vi "TestStand_Control ( Configure_Application_Manager ).vi"(8 "error IO":errorcluster, 11 "TestStand UI Data":T1) -> (0 "error IO 2":errorcluster, 3 "TestStand UI Data 2":T1)   [LabVIEW 2018, in "TestStand_Control.lvlib"]
uses:
  TestStand_Control.lvlib
  Module_Controls/TestStand UI Data.ctl
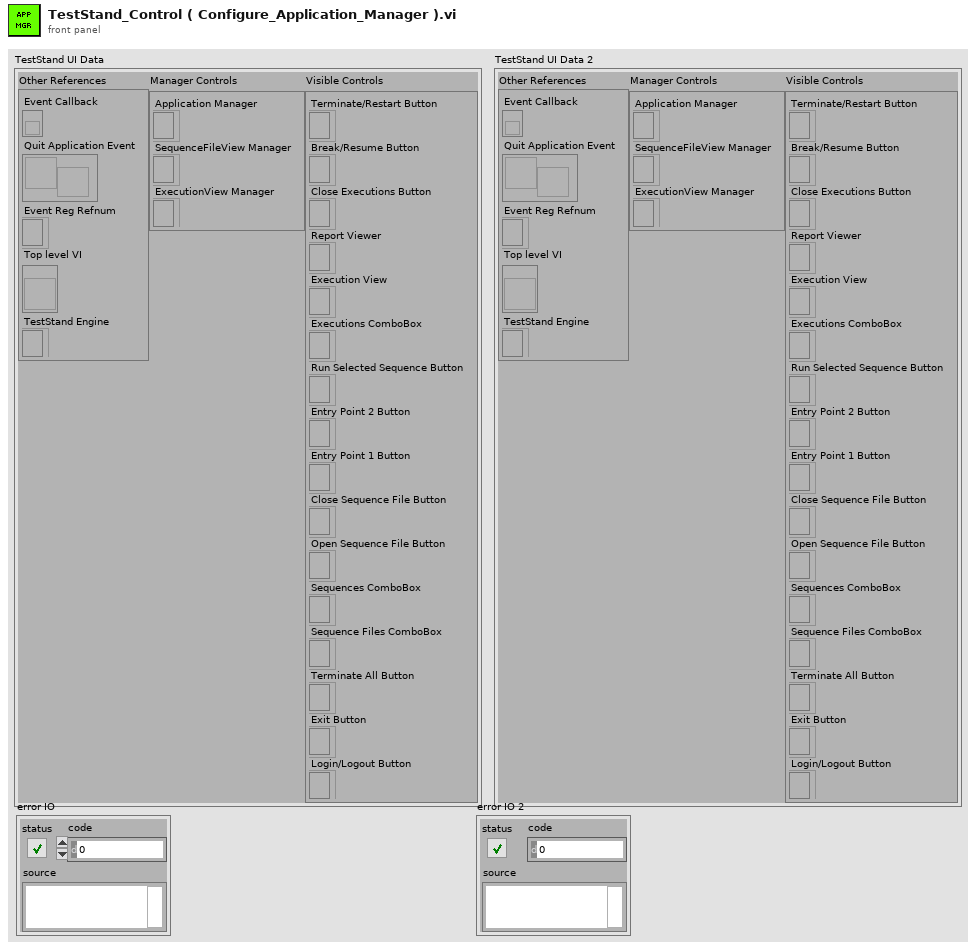
[diagram p1: front panel]
types:
  T1 = typedef "TestStand_Control.lvlib/TestStand UI Data.ctl" = cluster{"Other References":cluster{"Event Callback":refnum<k27>, "Quit Application Event":refnum<user-event>, "Event Reg Refnum":refnum<event-registration>, "Top level VI":refnum<vi>, "TestStand Engine":refnum<k7>}, "Manager Controls":cluster{"Application Manager":refnum<k7>, "SequenceFileView Manager":refnum<k7>, "ExecutionView Manager":refnum<k7>}, "Visible Controls":cluster{"Terminate/Restart Button":refnum<k7>, "Break/Resume Button":refnum<k7>, "Close Executions Button":refnum<k7>, "Report Viewer":refnum<k7>, "Execution View":refnum<k7>, "Executions ComboBox":refnum<k7>, "Run Selected Sequence Button":refnum<k7>, "Entry Point 2 Button":refnum<k7>, "Entry Point 1 Button":refnum<k7>, "Close Sequence File Button":refnum<k7>, "Open Sequence File Button":refnum<k7>, "Sequences ComboBox":refnum<k7>, "Sequence Files ComboBox":refnum<k7>, "Terminate All Button":refnum<k7>, "Exit Button":refnum<k7>, "Login/Logout Button":refnum<k7>}}
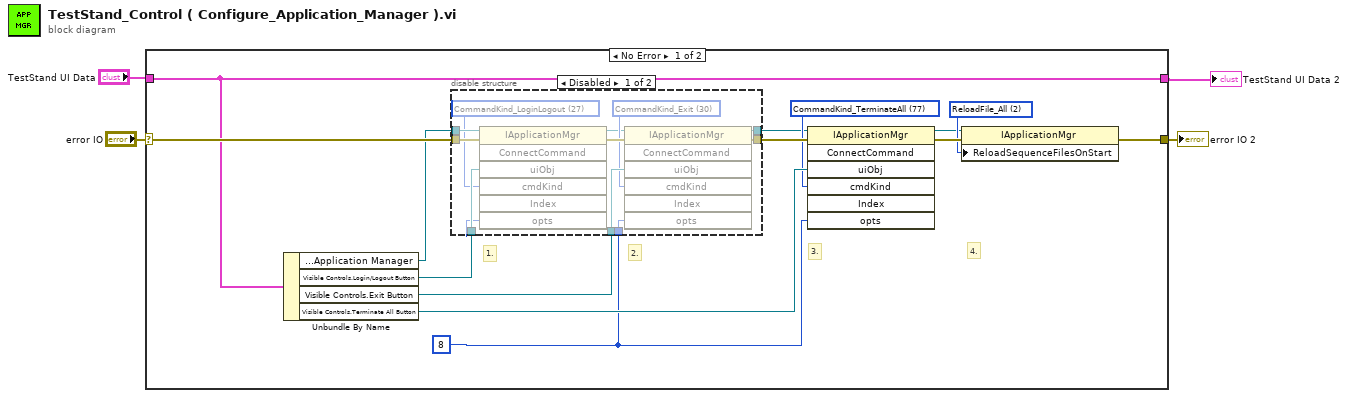
[diagram p0: block diagram]
diagram:
  n1 = case shown="No Error" "error IO" {
    selector: "error IO" -> [w18 w33]
    tunnel: [w12 w33] -> w1
    tunnel: "TestStand UI Data" -> [w9 w32]
    tunnel: [w9 w32] -> w3
    frame No Error {
      w6 = 77 items=["CommandKind_NotACommand"=0, "CommandKind_Container"=1, "CommandKind_Separator"=2, "CommandKind_Custom"=3, "CommandKind_OpenSequenceFile"=20, "CommandKind_Close"=21, "CommandKind_CloseAll"=22, "CommandKind_CloseCompletedExecutions"=23, "CommandKind_OpenWorkspaceBrowser"=24, "CommandKind_Login"=25, "CommandKind_Logout"=26, "CommandKind_LoginLogout"=27, "CommandKind_UnloadAllModules"=28, "CommandKind_MRUFile"=29, "CommandKind_Exit"=30, "CommandKind_Restart"=40, "CommandKind_RunEntryPoint"=41, "CommandKind_RunEntryPointOnSelectedSteps"=42, "CommandKind_LoopEntryPointOnSelectedSteps"=43, "CommandKind_RunCurrentSequence"=44, "CommandKind_RunSpecificSequence"=45, "CommandKind_RunSelectedSteps"=46, "CommandKind_RunSelectedStepsUsingEntryPointsSubmenu"=47, "CommandKind_LoopOnSelectedSteps"=48, "CommandKind_LoopOnSelectedStepsUsingEntryPointsSubmenu"=49, "CommandKind_BreakOnFirstStep"=50, "CommandKind_BreakOnStepFailure"=51, "CommandKind_BreakOnSequenceFailure"=52, "CommandKind_TracingEnabled"=53, "CommandKind_ToggleBreakpoint"=60, "CommandKind_SetRunModeSubmenu"=61, "CommandKind_RunModeForcePass"=62, "CommandKind_RunModeForceFail"=63, "CommandKind_RunModeSkip"=64, "CommandKind_RunModeNormal"=65, "CommandKind_Resume"=66, "CommandKind_StepInto"=67, "CommandKind_StepOver"=68, "CommandKind_StepOut"=69, "CommandKind_SetNextStep"=70, "CommandKind_Break"=71, "CommandKind_BreakResume"=72, "CommandKind_Terminate"=73, "CommandKind_TerminateRestart"=74, "CommandKind_Abort"=75, "CommandKind_BreakAll"=76, "CommandKind_TerminateAll"=77, "CommandKind_AbortAll"=78, "CommandKind_ResumeAll"=79, "CommandKind_DisplayBreakpointsAndWatchExpressions"=80, "CommandKind_DisplayBreakpointSettings"=81, "CommandKind_BreakpointSubmenu"=85, "CommandKind_ConfigureAdapters"=90, "CommandKind_ConfigureStationOptions"=91, "CommandKind_ConfigureSearchDirectories"=92, "CommandKind_ConfigureExternalViewers"=93, "CommandKind_ToolItem"=100, "CommandKind_CustomizeTools"=101, "CommandKind_ExecutionEntryPointInsertionMarker"=110, "CommandKind_ExecutionEntryPointDefaultMenuInsertionMarker"=111, "CommandKind_ConfigurationEntryPointInsertionMarker"=112, "CommandKind_ConfigurationEntryPointDefaultMenuInsertionMarker"=113, "CommandKind_DefaultFileMenu_Set"=120, "CommandKind_DefaultExecuteMenu_Set"=121, "CommandKind_DefaultDebugMenu_Set"=123, "CommandKind_DefaultConfigureMenu_Set"=124, "CommandKind_DefaultToolsMenu_Set"=125, "CommandKind_DefaultSequenceViewContextMenu_Set"=126, "CommandKind_DefaultListBarContextMenu_Set"=127, "CommandKind_MRUFiles_Set"=140, "CommandKind_ExecutionEntryPoints_Set"=141, "CommandKind_RunSequences_Set"=142, "CommandKind_RunSelectedStepsUsingEntryPoints_Set"=143, "CommandKind_LoopOnSelectedStepsUsingEntryPoints_Set"=144, "CommandKind_ConfigurationEntryPoints_Set"=145, "CommandKind_Tools_Set"=146] ("cmdKind")
      w8 = 8 ("opts")
      w13 = 2 items=["ReloadFile_None", "ReloadFile_Selected", "ReloadFile_All"] ("ReloadSequenceFilesOnStart")
      # "4."
      # "3."
      # "2."
      # "1."
      n2 = Unbundle By Name(w9) -> ("Manager Controls.Application Manager"=w11:refnum<k7>, "Visible Controls.Login/Logout Button"=w17:refnum<k7>, "Visible Controls.Exit Button"=w16:refnum<k7>, "Visible Controls.Terminate All Button"=w15:refnum<k7>)
      n3 = disable-structure shown="Disabled" {
        disable-tunnel: w18 -> [w29 w30]
        disable-tunnel: w17 -> [w28 _]
        disable-tunnel: w16 -> [w27 _]
        disable-tunnel: w11 -> [w26 w31]
        disable-tunnel: w8 -> [w25 _]
        disable-tunnel: [w23 w30] -> w7
        disable-tunnel: [w20 w31] -> w5
        frame Disabled {
          w21 = 30 items=["CommandKind_NotACommand"=0, "CommandKind_Container"=1, "CommandKind_Separator"=2, "CommandKind_Custom"=3, "CommandKind_OpenSequenceFile"=20, "CommandKind_Close"=21, "CommandKind_CloseAll"=22, "CommandKind_CloseCompletedExecutions"=23, "CommandKind_OpenWorkspaceBrowser"=24, "CommandKind_Login"=25, "CommandKind_Logout"=26, "CommandKind_LoginLogout"=27, "CommandKind_UnloadAllModules"=28, "CommandKind_MRUFile"=29, "CommandKind_Exit"=30, "CommandKind_Restart"=40, "CommandKind_RunEntryPoint"=41, "CommandKind_RunEntryPointOnSelectedSteps"=42, "CommandKind_LoopEntryPointOnSelectedSteps"=43, "CommandKind_RunCurrentSequence"=44, "CommandKind_RunSpecificSequence"=45, "CommandKind_RunSelectedSteps"=46, "CommandKind_RunSelectedStepsUsingEntryPointsSubmenu"=47, "CommandKind_LoopOnSelectedSteps"=48, "CommandKind_LoopOnSelectedStepsUsingEntryPointsSubmenu"=49, "CommandKind_BreakOnFirstStep"=50, "CommandKind_BreakOnStepFailure"=51, "CommandKind_BreakOnSequenceFailure"=52, "CommandKind_TracingEnabled"=53, "CommandKind_ToggleBreakpoint"=60, "CommandKind_SetRunModeSubmenu"=61, "CommandKind_RunModeForcePass"=62, "CommandKind_RunModeForceFail"=63, "CommandKind_RunModeSkip"=64, "CommandKind_RunModeNormal"=65, "CommandKind_Resume"=66, "CommandKind_StepInto"=67, "CommandKind_StepOver"=68, "CommandKind_StepOut"=69, "CommandKind_SetNextStep"=70, "CommandKind_Break"=71, "CommandKind_BreakResume"=72, "CommandKind_Terminate"=73, "CommandKind_TerminateRestart"=74, "CommandKind_Abort"=75, "CommandKind_BreakAll"=76, "CommandKind_TerminateAll"=77, "CommandKind_AbortAll"=78, "CommandKind_ResumeAll"=79, "CommandKind_DisplayBreakpointsAndWatchExpressions"=80, "CommandKind_DisplayBreakpointSettings"=81, "CommandKind_BreakpointSubmenu"=85, "CommandKind_ConfigureAdapters"=90, "CommandKind_ConfigureStationOptions"=91, "CommandKind_ConfigureSearchDirectories"=92, "CommandKind_ConfigureExternalViewers"=93, "CommandKind_ToolItem"=100, "CommandKind_CustomizeTools"=101, "CommandKind_ExecutionEntryPointInsertionMarker"=110, "CommandKind_ExecutionEntryPointDefaultMenuInsertionMarker"=111, "CommandKind_ConfigurationEntryPointInsertionMarker"=112, "CommandKind_ConfigurationEntryPointDefaultMenuInsertionMarker"=113, "CommandKind_DefaultFileMenu_Set"=120, "CommandKind_DefaultExecuteMenu_Set"=121, "CommandKind_DefaultDebugMenu_Set"=123, "CommandKind_DefaultConfigureMenu_Set"=124, "CommandKind_DefaultToolsMenu_Set"=125, "CommandKind_DefaultSequenceViewContextMenu_Set"=126, "CommandKind_DefaultListBarContextMenu_Set"=127, "CommandKind_MRUFiles_Set"=140, "CommandKind_ExecutionEntryPoints_Set"=141, "CommandKind_RunSequences_Set"=142, "CommandKind_RunSelectedStepsUsingEntryPoints_Set"=143, "CommandKind_LoopOnSelectedStepsUsingEntryPoints_Set"=144, "CommandKind_ConfigurationEntryPoints_Set"=145, "CommandKind_Tools_Set"=146] ("cmdKind")
          w22 = 27 items=["CommandKind_NotACommand"=0, "CommandKind_Container"=1, "CommandKind_Separator"=2, "CommandKind_Custom"=3, "CommandKind_OpenSequenceFile"=20, "CommandKind_Close"=21, "CommandKind_CloseAll"=22, "CommandKind_CloseCompletedExecutions"=23, "CommandKind_OpenWorkspaceBrowser"=24, "CommandKind_Login"=25, "CommandKind_Logout"=26, "CommandKind_LoginLogout"=27, "CommandKind_UnloadAllModules"=28, "CommandKind_MRUFile"=29, "CommandKind_Exit"=30, "CommandKind_Restart"=40, "CommandKind_RunEntryPoint"=41, "CommandKind_RunEntryPointOnSelectedSteps"=42, "CommandKind_LoopEntryPointOnSelectedSteps"=43, "CommandKind_RunCurrentSequence"=44, "CommandKind_RunSpecificSequence"=45, "CommandKind_RunSelectedSteps"=46, "CommandKind_RunSelectedStepsUsingEntryPointsSubmenu"=47, "CommandKind_LoopOnSelectedSteps"=48, "CommandKind_LoopOnSelectedStepsUsingEntryPointsSubmenu"=49, "CommandKind_BreakOnFirstStep"=50, "CommandKind_BreakOnStepFailure"=51, "CommandKind_BreakOnSequenceFailure"=52, "CommandKind_TracingEnabled"=53, "CommandKind_ToggleBreakpoint"=60, "CommandKind_SetRunModeSubmenu"=61, "CommandKind_RunModeForcePass"=62, "CommandKind_RunModeForceFail"=63, "CommandKind_RunModeSkip"=64, "CommandKind_RunModeNormal"=65, "CommandKind_Resume"=66, "CommandKind_StepInto"=67, "CommandKind_StepOver"=68, "CommandKind_StepOut"=69, "CommandKind_SetNextStep"=70, "CommandKind_Break"=71, "CommandKind_BreakResume"=72, "CommandKind_Terminate"=73, "CommandKind_TerminateRestart"=74, "CommandKind_Abort"=75, "CommandKind_BreakAll"=76, "CommandKind_TerminateAll"=77, "CommandKind_AbortAll"=78, "CommandKind_ResumeAll"=79, "CommandKind_DisplayBreakpointsAndWatchExpressions"=80, "CommandKind_DisplayBreakpointSettings"=81, "CommandKind_BreakpointSubmenu"=85, "CommandKind_ConfigureAdapters"=90, "CommandKind_ConfigureStationOptions"=91, "CommandKind_ConfigureSearchDirectories"=92, "CommandKind_ConfigureExternalViewers"=93, "CommandKind_ToolItem"=100, "CommandKind_CustomizeTools"=101, "CommandKind_ExecutionEntryPointInsertionMarker"=110, "CommandKind_ExecutionEntryPointDefaultMenuInsertionMarker"=111, "CommandKind_ConfigurationEntryPointInsertionMarker"=112, "CommandKind_ConfigurationEntryPointDefaultMenuInsertionMarker"=113, "CommandKind_DefaultFileMenu_Set"=120, "CommandKind_DefaultExecuteMenu_Set"=121, "CommandKind_DefaultDebugMenu_Set"=123, "CommandKind_DefaultConfigureMenu_Set"=124, "CommandKind_DefaultToolsMenu_Set"=125, "CommandKind_DefaultSequenceViewContextMenu_Set"=126, "CommandKind_DefaultListBarContextMenu_Set"=127, "CommandKind_MRUFiles_Set"=140, "CommandKind_ExecutionEntryPoints_Set"=141, "CommandKind_RunSequences_Set"=142, "CommandKind_RunSelectedStepsUsingEntryPoints_Set"=143, "CommandKind_LoopOnSelectedStepsUsingEntryPoints_Set"=144, "CommandKind_ConfigurationEntryPoints_Set"=145, "CommandKind_Tools_Set"=146] ("cmdKind")
          n4 = invoke class="IApplicationMgr" method="ConnectCommand"(reference=w26, error in=w29, "uiObj"=w28, "cmdKind"=w22, "opts"=w25) -> (reference out=w19:refnum<k7>, error out=w24:errorcluster)  [unwired: 2 in, 5 out]
          n5 = invoke class="IApplicationMgr" method="ConnectCommand"(reference=w19, error in=w24, "uiObj"=w27, "cmdKind"=w21, "opts"=w25) -> (reference out=w20:refnum<k7>, error out=w23:errorcluster)  [unwired: 2 in, 5 out]
        }
        frame Enabled {
        }
      }
      n6 = invoke class="IApplicationMgr" method="ConnectCommand"(reference=w5, error in=w7, "uiObj"=w15, "cmdKind"=w6, "opts"=w8) -> (reference out=w10:refnum<k7>, error out=w14:errorcluster)  [unwired: 2 in, 5 out]
      n7 = property class="IApplicationMgr"(reference=w10, error in=w14, "ReloadSequenceFilesOnStart"=w13) -> (error out=w12:errorcluster)  [unwired: 1 out]
    }
    frame Error {
    }
  }
  "TestStand UI Data 2" <- w3
  "error IO 2" <- w1
